vi "copy.vi"() -> ()   [LabVIEW 2014]
doc: "I. Description:\nThis example demonstrates how to acquire a continuous amount of data (Waveform) using the DAQ device's internal clock.\n\nII. Instructions for Running:\n1. Create an analog input voltage channel.\n2. Set the rate for the sample clock. Additionally, define the sample mode to be continuous.\n3. Call the Start VI to start the acquisition.\n4. Read the waveform data in a loop until the user hits the stop button or an error occurs.\nNote: This example reads data from one or more channels and returns an array of data. Use the Index Array function to access an individual channel of data.\n5. Call the Clear Task VI to clear the Task.\n6. Use the popup dialog box to display an error if any.\n\nIV. I/O Connections Overview:\nMake sure your signal input terminal matches the Physical Channel I/O Control. For further connection information, refer to your hardware reference manual."
uses:
  <vilib>/Utility/error.llb/DialogType.ctl
  <vilib>/addons/Digital Filter Design/NI_DigFilterLicensed.lvlib
  <vilib>/measure/NI_MAPro.lvlib
  <vilib>/DAQmx/create/channels.llb/DAQmx Create Channel (AI-Voltage-Basic).vi
  <vilib>/DAQmx/configure/timing.llb/DAQmx Timing (Sample Clock).vi
  <vilib>/Analysis/NI_AAL_SigProc.lvlib
  <vilib>/measure/mamon.llb/Waveform Peak Detection for 1 Chan.vi
  <vilib>/addons/Digital Filter Design/Design.llb/DFD IIR Notch Peak Design by BW.vi
  <vilib>/addons/Digital Filter Design/Process.llb/DFD Filtering (Wfm NChan).vi
  <vilib>/DAQmx/read.llb/DAQmx Read (Analog 1D Wfm NChan NSamp).vi
  <vilib>/imath/engines/lvmath2/RunTimeEngine/BuiltInFunctions/length/NIMS_length(GV).vi
  <vilib>/imath/engines/lvmath2/RunTimeEngine/RangeToken/NIMS_Range_R2 - Integer.vi
  <vilib>/imath/engines/lvmath2/RunTimeEngine/CommandStatement/MC_CommandStatement_break.vi
  <vilib>/imath/engines/lvmath2/RunTimeEngine/VariableToken/NIMS_VariableToken_CondDefinedDefinedByReplace.vi
  <vilib>/imath/engines/lvmath2/RunTimeEngine/IndexRead/NIMS V(S).vi
  <vilib>/imath/engines/lvmath2/RunTimeEngine/IndexReplace/NIMS V(S)=S.vi
  <vilib>/imath/engines/lvmath2/RunTimeEngine/ErrorHandling/NIMS_Create Error From Enums.vi
  <vilib>/imath/engines/lvmath2/RunTimeEngine/BuiltInFunctions/is_empty/NIMS_is_empty(GM).vi
  <vilib>/imath/engines/lvmath2/RunTimeEngine/BuiltInFunctions/abs/NIMS_abs(signed).vi
  <vilib>/imath/engines/lvmath2/RunTimeEngine/RowToken/NIMS_RowToken_M_SorRV.vi
  <vilib>/imath/engines/lvmath2/RunTimeEngine/BuiltInFunctions/length/NIMS_length(GM).vi
  <vilib>/imath/engines/lvmath2/RunTimeEngine/IndexRead/NIMS M(S).vi
  <vilib>/imath/engines/lvmath2/RunTimeEngine/NodeEndStatement/NIMS_NodeEndStatement_Output.vi
  <vilib>/imath/engines/lvmath2/RunTimeEngine/ErrorHandling/NIMS_Finalize Error.vi
panel:
  in  "peak detector width":i32=3 min=3
  out "Signal Plot":cluster{"Locations":dbl[], "Amplitudes":dbl[]}[](graph)
  in  "Stop":bool
  out "peaks found":i32
  out "valleys found":i32
  in  "PD width":i32=3 min=3
  in  "threshold":dbl format="%0.2f"
  out "#Peaks Found\n in 2 sec":i32
  out "ECG":waveform(dbl)(graph)
  out "Heart Rate \n(beats/min)":dbl
  out "Sound":waveform(dbl)(graph)
  out "2 peaks found?":bool
  in  "Samples to Read":i32=1000
  in  "Physical Channel":tag="Dev1/ai0"
  in  "Minimum Value":dbl=-10.0 caption="Min (V)" format="%0.2f"
  in  "Maximum Value":dbl=10.0 caption="Max (V)" format="%0.2f"
  in  "stop":bool
  in  "Sample Rate":dbl=10000.0 caption="Sample Rate (Hz)" format="%0.2f"
  # "For instructions, select Help>>Show Context Help"
  # "Thresholding Parameters"
  # "Channel Parameters"
  # "Make sure your figures are all on the same scale!!"
  # "A/D\nconversion"
  # "Timing Parameters"
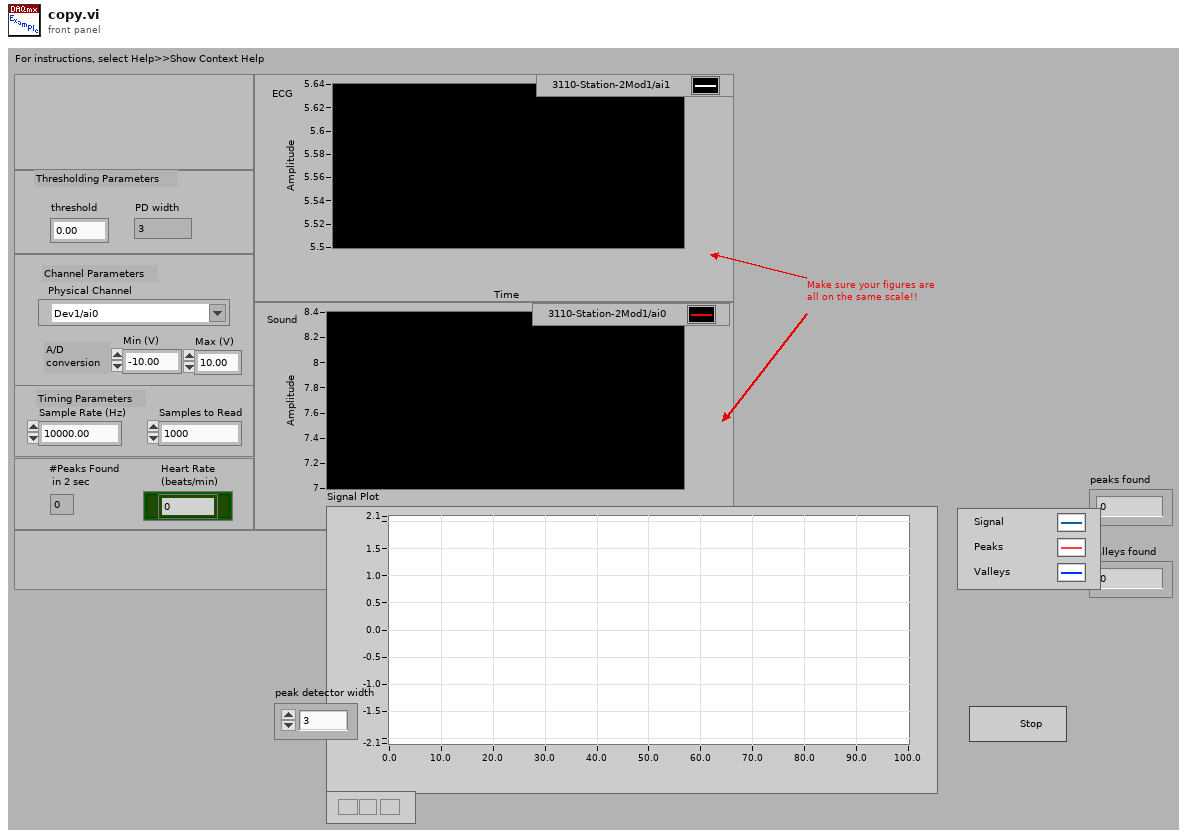
[diagram p1: front panel]
types:
  T1 = typedef "DialogType.ctl" = u16
  T2 = typedef "NI_DigFilterLicensed.lvlib/DFD Filter Obj.ctl" = cluster{"mSRate_Fs":dbl, "mSRate_Version":string, "mSRate_Comments":string, "mSRate_OrgCoef":T3, "mSRate_CurCoef":T3, "mSRate_Quantized?":bool, "mSRate_QCoef":T3, "mSRate_QSettings":T5[], "mSRate_Order":i32, "mSRate_Scaling":cluster{"mSRate_ScaleByPowerOf2?":bool, "mSRate_ScaleType":T7}}
  T3 = typedef "NI_DigFilterLicensed.lvlib/DFD Filter Coef.ctl" = cluster{"type":T4, "gain":dbl, "coef a (k)":dbl[], "coef b (v)":dbl[]}
  T4 = typedef "NI_DigFilterLicensed.lvlib/DFD Filter Structure Type Selector.ctl" = enum16{"Undefined", "FIR Direct Form", "FIR Direct Form Transposed", "FIR Symmetric", "FIR Antisymmetric", "IIR Direct Form I", "IIR Direct Form I Transposed", "IIR Direct Form II", "IIR Direct Form II Transposed", "IIR Cascaded Second Order Sections Form I", "IIR Cascaded Second Order Sections Form I Transposed", "IIR Cascaded Second Order Sections Form II", "IIR Cascaded Second Order Sections Form II Transposed", "Lattice Allpass (basic sections)", "Lattice Allpass (one multiplier sections)", "Lattice Allpass (normalized sections)", "Lattice AR (basic sections)", "Lattice AR (one multiplier sections)", "Lattice AR (normalized sections)", "Lattice MA (minimum phase)", "Lattice MA (maximum phase)", "Lattice ARMA (basic sections)", "Lattice ARMA (one multiplier sections)", "Lattice ARMA (normalized sections)"}
  T5 = typedef "NI_DigFilterLicensed.lvlib/dfd_Internal Quantization Settings.ctl" = cluster{"source":T6, "wl":i16, "iwl":i16, "overflow mode":enum16{"Saturation", "Wrap"}, "rounding mode":enum16{"Nearest", "Truncation"}, "signed?":bool}
  T6 = typedef "NI_DigFilterLicensed.lvlib/dfd_Internal Quantization Srcs.ctl" = u16
  T7 = typedef "NI_DigFilterLicensed.lvlib/DFD Coef Norm Type.ctl" = enum16{"No Norm", "Time Domain 1-Norm", "Time Domain 2-Norm", "Time Domain Inf-Norm"}
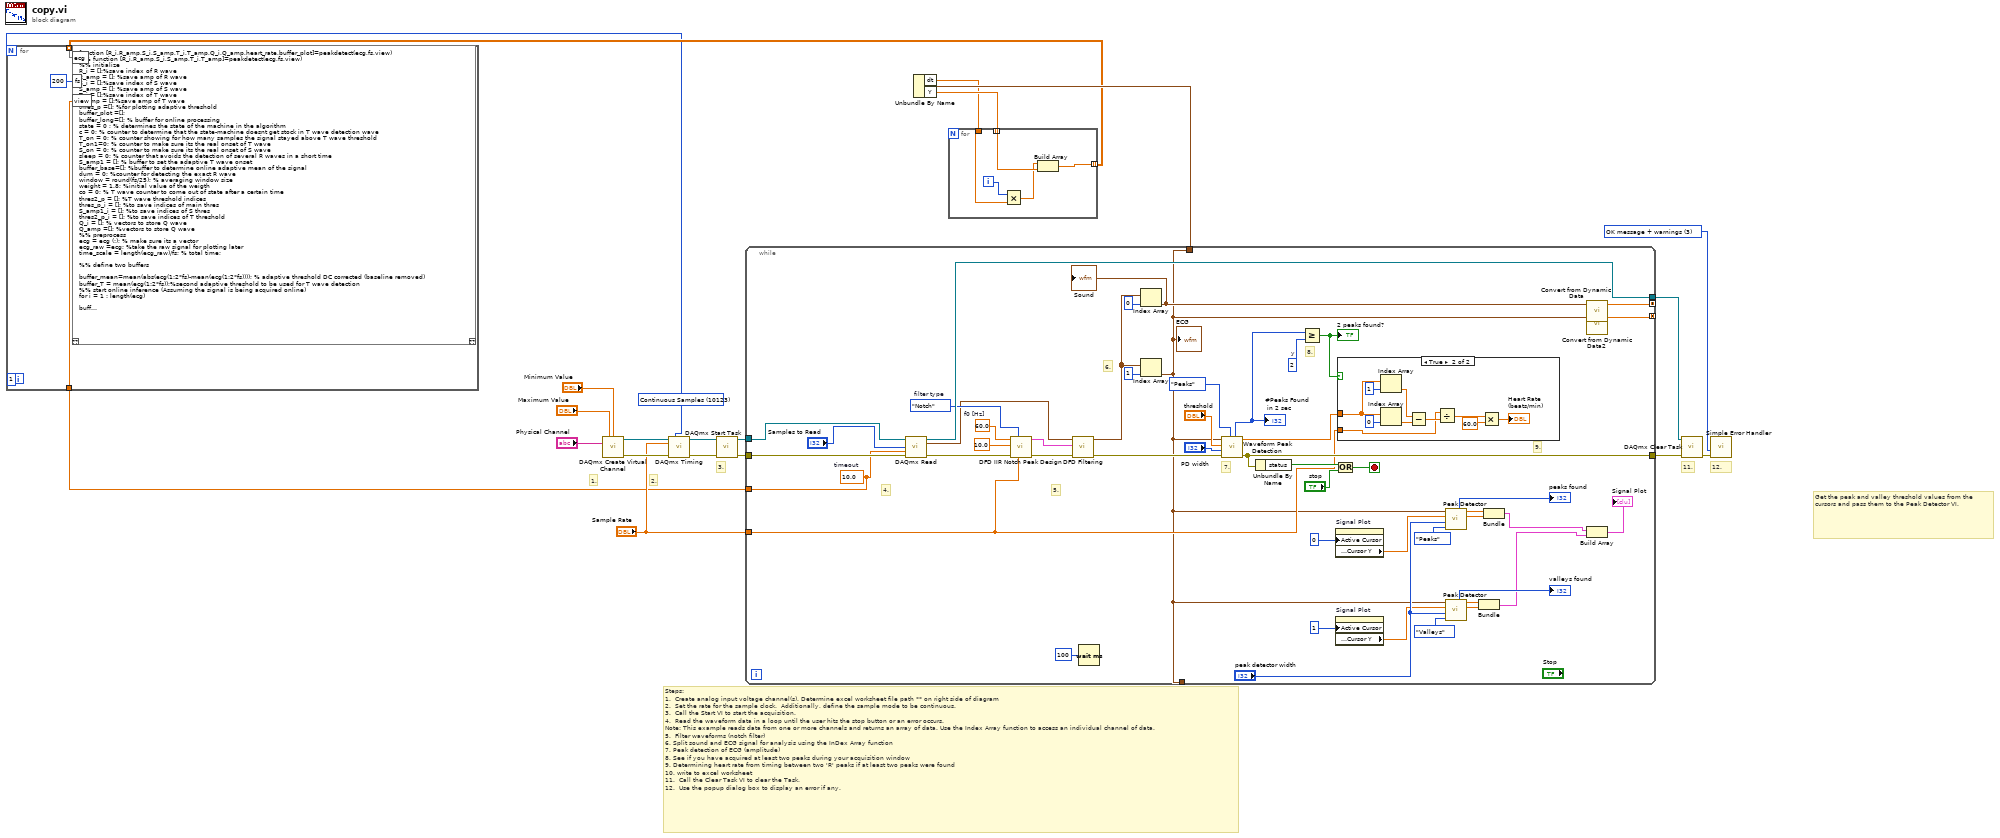
[diagram p0: block diagram]
diagram:
  w8 = T1 3 items=["no dialog", "OK message", "continue or stop message", "OK message + warnings", "continue/stop + warnings"] ("type of dialog (OK msg:1)")
  w1 = 10123 items=["Finite Samples"=10178, "Continuous Samples"=10123] ("sample mode")
  # "Get the peak and valley threshold values from the cursors and pass them to the Peak Detector VI."
  # "2."
  # "1."
  # "12."
  # "11."
  # "Steps: \n1.  Create analog input voltage channel(s). Determine excel worksheet file path ** on right side of diagram\n2.  Set the rate for the sample clock.  Additionally, define the sample mode to be continuous.\n3.  Call the Start VI to start the acquisition.\n4.  Read the waveform data in a loop until the user hits the stop button or an error occurs.\nNote: This example reads data from one or more channels and returns an array of data. Use the Index Array function to access an individual channel of data.\n5.  Filter waveforms (notch filter)\n6. Split sound and ECG signal for analysis using the InDex Array function\n7. Peak detection of ECG (amplitude)\n8. See if you have acquired at least two peaks during your acquisition window\n9. Determining heart rate from timing between two 'R' peaks if at least two peaks were found\n10. write to excel worksheet\n11.  Call the Clear Task VI to clear the Task.\n12.  Use the popup dialog box to display an error if any."
  # "3."
  n1 = call-poly <vilib>:"DAQmx Create Virtual Channel.vi"("maximum value"="Maximum Value", "minimum value"="Minimum Value", "physical channels"="Physical Channel") -> ("task out"=w15:refnum<k21>, "error out"=w18:errorcluster)  [unwired: 6 in, 5 out]
  n2 = call-poly <vilib>:"DAQmx Timing.vi"("task/channels in"=w15, "sample mode"=w1, "rate"="Sample Rate", "error in"=w18) -> ("task out"=w11:refnum<k21>, "error out"=w10:errorcluster)  [unwired: 3 in, 7 out]
  n3 = call <vilib>:"DAQmx Start Task.vi"("task/channels in"=w11, "error in"=w10) -> ("task out"=w14:refnum<k21>, "error out"=w17:errorcluster)  [unwired: 12 out]
  n4 = while {
    tunnel: w17 -> [w69]
    tunnel: w14 -> [w68]
    tunnel: [w67] -> w13
    tunnel: [w46] -> w9
    tunnel: "Sample Rate" -> [w42]
    tunnel: [w41] -> _ mode=concatenating
    tunnel: [w40] -> _ mode=concatenating
    tunnel: [w22] -> _
    tunnel: [w22] -> w5
    tunnel: [w21] -> w2
    stop <- w65 stop-if-true
    w44 = 2  # y
    w60 = enum16{"Notch", "Peak"}."Notch"  # filter type
    w61 = 60.0  # f0 [Hz]
    w21 = 10.0  # timeout
    # "9."
    # "8."
    # "7."
    # "6."
    # "5."
    # "4."
    n5 = call-poly <vilib>:"DAQmx Read.vi"("task/channels in"=w68, "number of samples per channel"="Samples to Read", "timeout"=w21, "error in"=w69) -> ("task out"=w67:refnum<k21>, "data"=w51:waveform(dbl)[], "error out"=w58:errorcluster)  [unwired: 9 out]
    n6 = call-poly <vilib>:"DFD IIR Notch Peak Design.vi"("fs [Hz]"=w42, "filter type"=w60, "error in (no error)"=w58, "Df [Hz]"=10.0 ("Q factor"), "f0 [Hz]"=w61) -> ("error out"=w57:errorcluster, "filter out"=w59:T2)  [unwired: 1 in, 4 out]
    n7 = call-poly <vilib>:"DFD Filtering.vi"("error in (no error)"=w57, "filter"=w59, "signal in"=w51) -> ("error out"=w47:errorcluster, "signal out"=w48:waveform(dbl)[])  [unwired: 1 in, 6 out]
    n8 = Wait (ms)(milliseconds to wait=u32 100) -> ()  [unwired: 1 out]
    n9 = Index Array(array=w48, index=0) -> (element=w50:waveform(dbl))
    "Sound" <- w50
    n10 = Index Array(array=w48, index=1) -> (element=w22:waveform(dbl))
    "ECG" <- w22
    n11 = call-poly <vilib>:"Waveform Peak Detection.vi"("peaks/valleys"=enum32{"Peaks", "Valleys"}."Peaks", "error in"=w47, "width"="PD width", "threshold"="threshold", "Signal In"=w22) -> ("error out"=w46:errorcluster, "Locations"=w56:dbl[], "# found"=w45:i32)  [unwired: 2 in, 2 out]
    "#Peaks Found\n in 2 sec" <- w45
    n12 = Unbundle By Name(w46) -> ("status"=w66:bool)
    n13 = Greater Or Equal?(x=w45, y=w44) -> (x >= y?=w43:bool)
    "2 peaks found?" <- w43
    n14 = Or(x=w66, y="stop") -> (x .or. y?=w65:bool)
    n15 = property on="Signal Plot" class="XYGraph (strict)"("Active Cursor"=u32 0) -> ("Cursor.Cursor Position:Cursor Y"=w33:dbl)  [unwired: 2 in, 2 out]
    n16 = property on="Signal Plot" class="XYGraph (strict)"("Active Cursor"=u32 1) -> ("Cursor.Cursor Position:Cursor Y"=w34:dbl)  [unwired: 2 in, 2 out]
    n17 = case shown="True" w43 {
      tunnel: w56 -> [_ w74]
      tunnel: w42 -> [_ w70]
      frame False {
      }
      frame True {
        n18 = Index Array(array=w74, index=1) -> (element=w76:dbl)
        n19 = Index Array(array=w74, index=0) -> (element=w75:dbl)
        n20 = Subtract(x=w76, y=w75) -> (x-y=w71:dbl)
        n21 = Divide(x=w70, y=w71) -> (x/y=w77:dbl)
        n22 = Multiply(x=w77, y=60.0) -> (x*y=→"Heart Rate \n(beats/min)":dbl)
      }
    }
    n23 = call <vilib>:"Peak Detector.vi"("peaks/valleys"=enum32{"Peaks", "Valleys"}."Peaks", "width"="peak detector width", "threshold"=w33, "X"=w22) -> ("Amplitudes"=w27:dbl[], "Locations"=w31:dbl[], "# found"=→"peaks found":i32)  [unwired: 3 in, 2 out]
    n24 = call <vilib>:"Peak Detector.vi"("peaks/valleys"=enum32{"Peaks", "Valleys"}."Valleys", "width"="peak detector width", "threshold"=w34, "X"=w22) -> ("Amplitudes"=w29:dbl[], "Locations"=w28:dbl[], "# found"=→"valleys found":i32)  [unwired: 3 in, 2 out]
    n25 = Bundle("Locations"=w28, "Amplitudes"=w29) -> (w23:cluster{"Locations":dbl[], "Amplitudes":dbl[]})  [unwired: 1 in]
    n26 = Bundle("Locations"=w31, "Amplitudes"=w27) -> (w24:cluster{"Locations":dbl[], "Amplitudes":dbl[]})  [unwired: 1 in]
    n27 = call "Convert from Dynamic Data"("Dynamic Data Type"=w50) -> ("Array"=w41:dbl[])  [unwired: 3 out]
    n28 = call "Convert from Dynamic Data2"("Dynamic Data Type"=w22) -> ("Array"=w40:dbl[])  [unwired: 3 out]
    n29 = Build Array(w24, w23) -> (→"Signal Plot":cluster{"Locations":dbl[], "Amplitudes":dbl[]}[])
  }
  n30 = Unbundle By Name(w5) -> ("dt"=w4:dbl, "Y"=w6:dbl[])
  n31 = for {
    tunnel: w6 -> [w84] mode=indexing
    tunnel: [w83] -> w3 mode=indexing
    tunnel: w4 -> [w82]
    i -> [w81]
    n32 = Multiply(x=w81, y=w82) -> (x*y=w80:dbl)
    n33 = Build Array(w80, w84) -> (w83:dbl[])
  }
  n34 = for {
    N: w1 -> [_]
    tunnel: w3 -> [w87] mode=indexing
    tunnel: w2 -> [w85]
    (unwired) 1
    n35 = mathscript code="function [R_i,R_amp,S_i,S_amp,T_i,T_amp,Q_i,Q_amp,heart_rate,buffer_plot]=peakdetect(ecg,fs,view)\n%% function [R_i,R_amp,S_i,S_amp,T_i,T_amp]=peakdetect(ecg,fs,view)\n%% initialize\nR_i = [];%save index of R wave\nR_amp = []; %save amp of R wave\nS_i = [];%save index of S wave\nS_amp = []; %save amp of S wave\nT_i = [];%save index of T wave\nT_amp = [];%save amp of T wave\nthres_p =[]; %for plotting adaptive threshold\nbuffer_plot =[];\nbuffer_long=[]; % buffer for online processing\nstate = 0 ; % determines the state of the machine in the algorithm\nc = 0; % counter to determine that the state-machine doesnt get stock in T wave detection wave\nT_on = 0; % counter showing for how many samples the signal stayed above T wave threshold\nT_on1=0; % counter to make sure its the real onset of T wave\nS_on = 0; % counter to make sure its the real onset of S wave\nsleep = 0; % counter that avoids the detection of several R waves in a short time\nS_amp1 = []; % buffer to set the adaptive T wave onset\nbuffer_base=[]; %buffer to determine online adaptive mean of the signal\ndum = 0; %counter for detecting the exact R wave\nwindow = round(fs/25); % averaging window size\nweight = 1.8; %initial value of the weigth\nco = 0; % T wave counter to come out of state after a certain time\nthres2_p = []; %T wave threshold indices\nthres_p_i = []; %to save indices of main thres\nS_amp1_i = []; %to save indices of S thres\nthres2_p_i = []; %to save indices of T threshold\nQ_i = []; % vectors to store Q wave\nQ_amp =[]; %vectors to store Q wave\n%% preprocess\necg = ecg (:); % make sure its a vector\necg_raw =ecg; %take the raw signal for plotting later\ntime_scale = length(ecg_raw)/fs; % total time;\n\n%% define two buffers\n\nbuffer_mean=mean(abs(ecg(1:2*fs)-mean(ecg(1:2*fs)))); % adaptive threshold DC corrected (baseline removed)\nbuffer_T = mean(ecg(1:2*fs));%second adaptive threshold to be used for T wave detection\n%% start online inference (Assuming the signal is being acquired online)\nfor i = 1 : length(ecg)\n    \nbuffer_long = [buffer_long ecg(i)] ; % save the upcoming new samples\nbuffer_base = [buffer_base ecg(i)] ; % save the baseline samples\n\n%% Renew the mean and adapt it to the signal after 1 second of processing\nif length(buffer_base) >= 2*fs\n    buffer_mean = mean(abs(buffer_base(1:2*fs)-mean(buffer_base(1:2*fs))));\n    buffer_T = mean(buffer_base(1:2*fs));\n    buffer_base =[];\nend\n\n%% smooth the signal by taking the average of 15 samples and add the new upcoming samples\n  if length(buffer_long)>= window % take a window with length 15 samples for averaging\n      mean_online = mean(buffer_long);  % take the mean\n      buffer_plot =[buffer_plot mean_online]; % save the processed signal\n      \n      \n    %% Enter state 1(putative R wave) as soon as that the mean exceeds the double time of threshold  \n    if state == 0  \n     if length(buffer_plot) >= 3   %added to handle bugg for now\n      if mean_online > buffer_mean*weight && buffer_plot(i-1-window) > buffer_plot(i-window)    %2.4*buffer_mean   \n          state = 1; % entered R peak detection mode\n          currentmax = buffer_plot(i-1-window);\n          ind = i-1-window;\n          thres_p = [thres_p buffer_mean*weight];\n          thres_p_i = [thres_p_i ind];\n      else     \n          state = 0;\n      end\n     end\n    end\n    \n    %% Locate the R wave location by finding the highest local maxima\n      if state == 1 % look for the highest peak\n          \n            if  currentmax > buffer_plot(i-window)\n                dum = dum + 1;\n                if dum > 4 \n                R_i = [R_i ind];%save index\n                R_amp = [R_amp buffer_plot(ind)]; %save index\n                % Locate Q wave\n                [Q_tamp Q_ti] = min(buffer_plot(ind-round(0.040*fs):(ind)));\n                Q_ti = ind-round(0.040*fs) + Q_ti -1;\n                Q_i = [Q_i Q_ti];\n                Q_amp = [Q_amp Q_tamp];\n                \n                \n                if length(R_amp) > 8\n                weight = 0.30*mean(R_amp(end-7:end)); %calculate the 35% of the last 8 R waves\n                weight = weight/buffer_mean;\n                end\n                state = 2; % enter S detection mode state 2\n                dum = 0;\n                end\n            else\n                dum = 0;\n                state = 0;\n            end \n            \n      end\n      \n    %% check weather the signal drops below the threshold to look for S wave\n      if state == 2 \n        if  mean_online <= buffer_mean     % check the threshold\n             state = 3;   %enter S detection           \n        end\n      end\n      \n      %% Enter S wave detection state3 (S detection)\n          if state == 3\n            co = co + 1; \n            \n          if co < round(0.200*fs)\n            if buffer_plot(i-window-1) <= buffer_plot(i-window) % see when the slope changes\n             S_on = S_on + 1; % set a counter to see if its a real change or just noise\n             if S_on >= round(0.0120*fs)\n             S_i = [S_i i-window-4];%save index of S wave\n             S_amp = [S_amp buffer_plot(i-window-4)];%save index\n             S_amp1 = [S_amp1  buffer_plot(i-window-4)]; %ecg(i-4)\n             S_amp1_i = [S_amp1_i ind]; %index of S_amp1_i\n             state = 4; % enter T detection mode\n             S_on = 0;\n             co = 0;\n             end\n            end\n          else\n              state = 4;\n              co = 0;\n          end\n          end\n      \n       %% enter state 4 possible T wave detection\n       if state == 4    \n         if mean_online < buffer_mean % see if the signal drops below mean \n           state = 6; % confirm\n         end\n       end\n       %% Enter state 6 which is T wave possible detection\n       if state ==6   \n         c = c + 1; % set a counter to exit the state if no T wave detected after 0.3 second\n         if c <= 0.7*fs  \n             % set a double threshold based on the last detected S wave and\n             % baseline of the signal and look for T wave in between these\n             % two threshold\n             thres2 = ((abs(abs(buffer_T)-abs(S_amp1(end))))*3/4 + S_amp1(end)); \n             thres2_p =[thres2_p thres2];\n             thres2_p_i =[thres2_p_i ind];\n             if mean_online > thres2\n              T_on = T_on +1; % make sure it stays on for at least 3 samples\n              if T_on >= round(0.0120*fs)\n               if buffer_plot(i-window-1)>= buffer_plot(i-window)\n                   T_on1 = T_on1+1; % make sure its a real slope change\n                  if T_on1 > round(0.0320*fs) \n                   T_i = [T_i i-window-11];%save index of T wave\n                   T_amp = [T_amp  buffer_plot(i-window-11)];%save index\n                   state = 5; % enter sleep mode\n                   T_on = 0;\n                   T_on1 = 0;\n                  end\n                                      \n               end\n              end\n             end\n             \n            \n          \n         else\n             state= 5; % enter Sleep mode\n         end\n         \n       end  \n      \n        \n       %% this state is for avoiding the detection of a highly variate noise or another peak\n       % this avoids detection of two peaks R waves less than half a second\n       if state==5\n           sleep =sleep+c+1;\n           c = 0;\n           if sleep/fs >= 0.400\n               state = 0;\n               sleep = 0;%look for the next peak\n           end  \n       end\n      \n      % update the online buffer by removing the oldest sample\n      buffer_long(1)=[];\n      \n      \n  end\n  \nend\n\n%% conditions\nR_R = diff(R_i); % calculate the distance between each R wave\n\n% compute the min max R-R wave\nmax_R_interval = max(R_R);\nmin_R_interval = min(R_R);"("fs"=200, "view"=w85, "ecg"=w87) -> ()  [unwired: 1 in, 1 out]
  }
  n36 = call <vilib>:"DAQmx Clear Task.vi"("task in"=w13, "error in"=w9) -> ("error out"=w16:errorcluster)  [unwired: 13 out]
  n37 = call <vilib>:"Simple Error Handler.vi"("type of dialog (OK msg:1)"=w8, "error in (no error)"=w16) -> ()  [unwired: 8 out]
